vi "Logging Message Loop.vi"(8 "error in (no error)":errorcluster, 10 "Data Queue":T1, 11 "Message Queues":T2) -> (0 "error out":errorcluster)   [LabVIEW 2015, in "Logging.lvlib"]
doc: "The message loop subVI to handle messages pertaining to logging data."
uses:
  Logging.lvlib
  Support VIs/Message Queue/All Message Queues.ctl
  Support VIs/Message Queue/Message Cluster.ctl
  controls/Data queue.ctl
  Acquisition/Generic data packet.ctl
  My Graphs/Gps Map Graph coordinates.ctl
  Logging Configuration.ctl
  Logging State.ctl
  Support VIs/Message Queue/Enqueue Message (Single).vi
  <vilib>/Utility/error.llb/Error Cluster From Error Code.vi
  <vilib>/ErrorRing/Error Ring.xnode
  Support VIs/Message Queue/Message Queue.lvlib
  Acquisition/Acquisition.lvlib
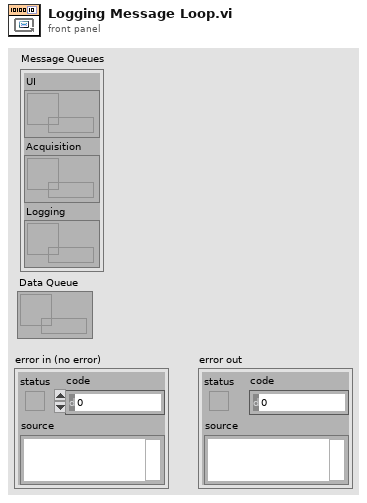
[diagram p1: front panel]
types:
  T1 = typedef "Data queue.ctl" = refnum<queue>
  T2 = typedef "Message Queue.lvlib/All Message Queues.ctl" = cluster{"UI":refnum<queue>, "Acquisition":refnum<queue>, "Logging":refnum<queue>}
  T3 = typedef "Logging.lvlib/Logging Configuration.ctl" = cluster{"Log File Base Path":path, "TDMS File Reference":refnum<k34>, "Data format":enum16{"IDRA data", "XAM data"}}
  T4 = cluster{"log_number":i32, "log_timestamp":string}
  T5 = typedef "Logging.lvlib/Logging State.ctl" = enum16{"Idle", "Logging"}
  T6 = enum16{"open", "open or create", "create or replace", "create", "open (read-only)"}
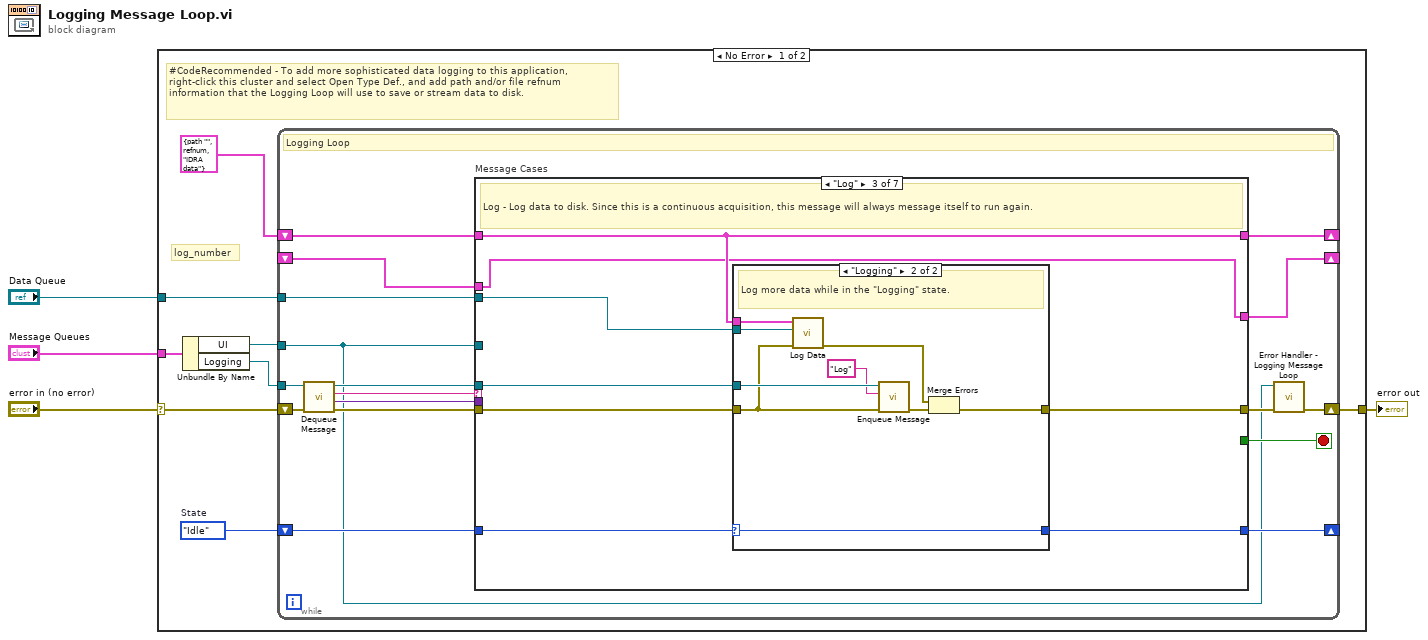
[diagram p0: block diagram]
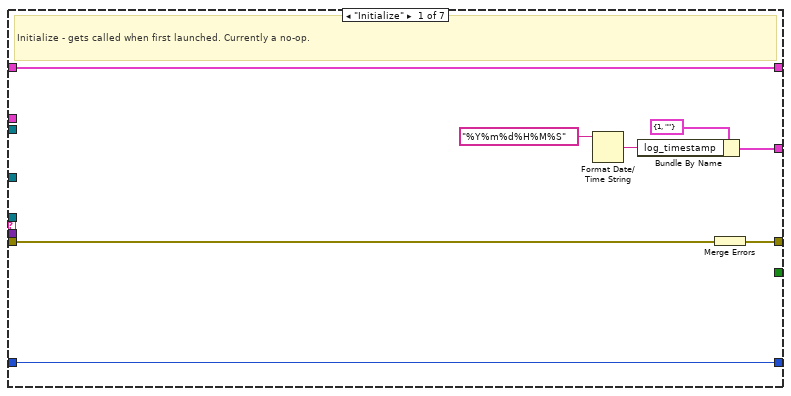
[diagram p2: hidden frame]
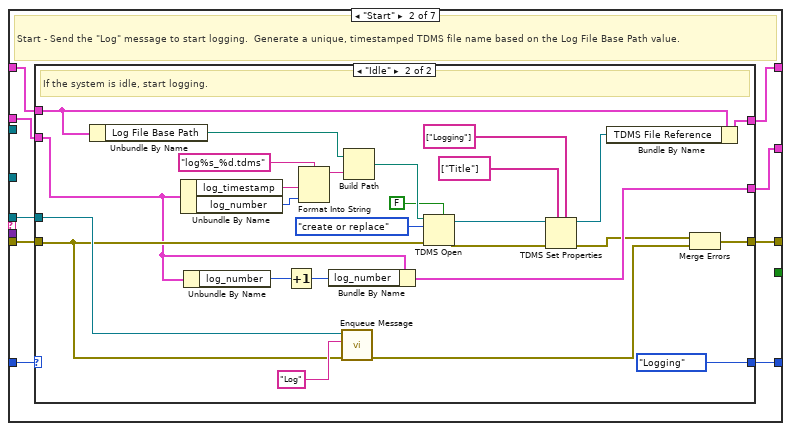
[diagram p3: hidden frame]
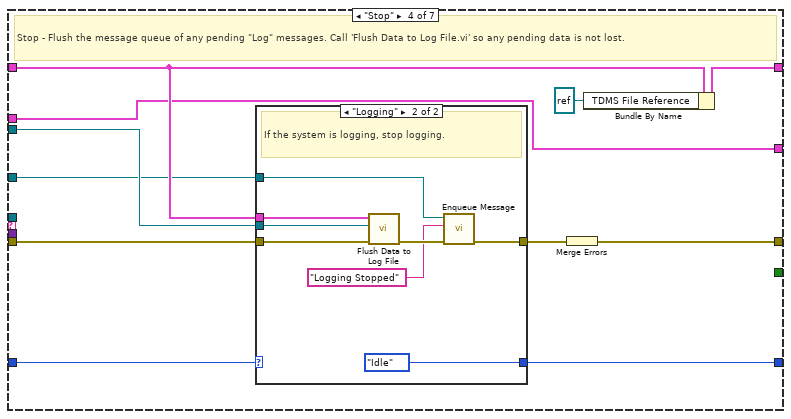
[diagram p6: hidden frame]
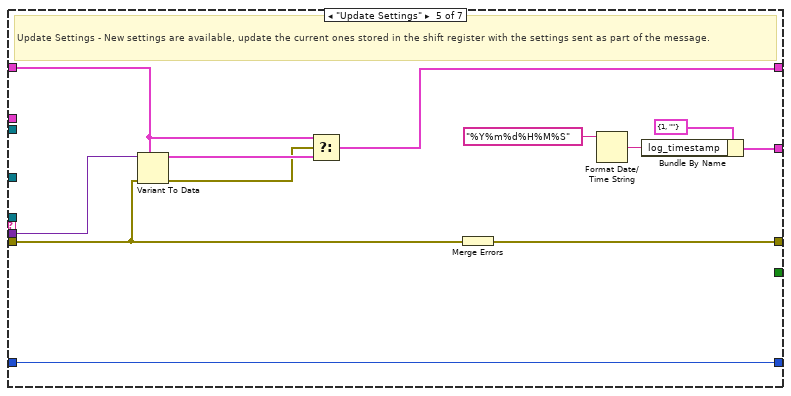
[diagram p8: hidden frame]
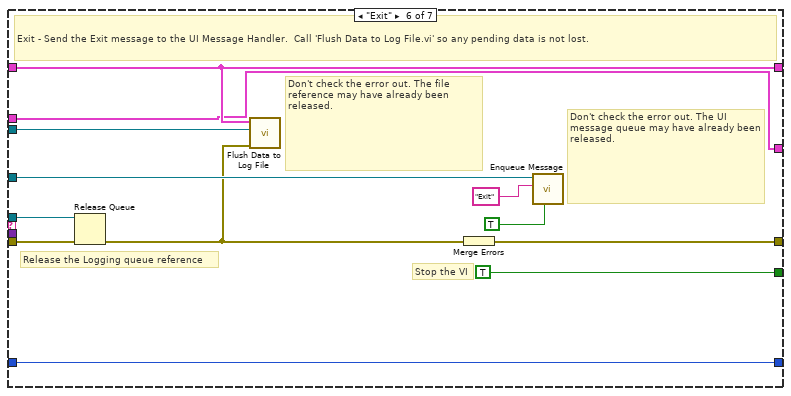
[diagram p9: hidden frame]
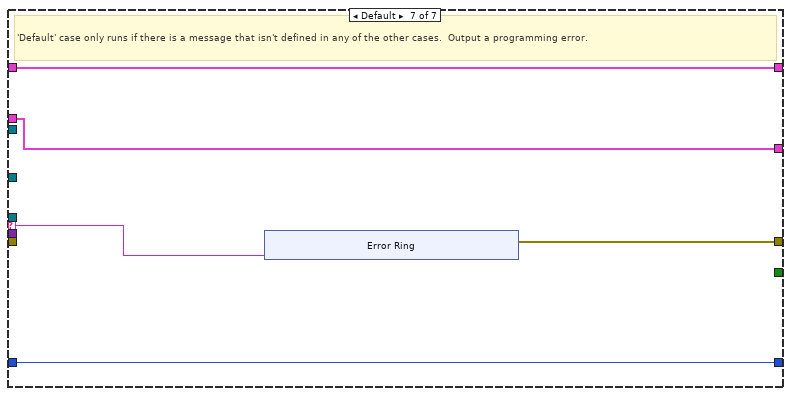
[diagram p10: hidden frame]
diagram:
  n1 = case shown="No Error" "error in (no error)" {
    selector: "error in (no error)" -> [w8 w153]
    tunnel: "Message Queues" -> [w12 _]
    tunnel: [w10 w153] -> w3
    tunnel: "Data Queue" -> [w7 _]
    frame No Error {
      w5 = Logging_State."Idle"  # State
      # "log_number"
      # "#CodeRecommended - To add more sophisticated data logging to this application, right-click this cluster and select Open Type Def., and add path and/or file refnum information that the Logging Loop will use to save or stream data to disk."
      n2 = Unbundle By Name(w12) -> ("UI"=w6:refnum<queue>, "Logging"=w11:refnum<queue>)
      n3 = while {
        tunnel: w11 -> [w21]
        shift-right: [w28] -> _
        shift-left: T3 {"Log File Base Path"=path "", "TDMS File Reference"=refnum, "Data format"=enum."IDRA data"} ("Logging Configuration") -> [w29]
        shift-right: [w17] -> w10
        shift-left: w8 -> [w26]
        tunnel: w6 -> [w15]
        tunnel: w7 -> [w20]
        shift-right: [w18] -> _
        shift-left: w5 -> [w19]
        shift-right: [w14] -> _
        shift-left: _ -> [w13]
        stop <- w27 stop-if-true
        # "Logging Loop"
        n4 = call "Dequeue Message.vi"("error in (no error)"=w26, "Message Queue"=w21) -> ("error out"=w25:errorcluster, "Message Data"=w23:variant, "Message"=w24:string, "dup Message Queue"=w22:refnum<queue>)  [unwired: 6 in]
        n5 = case "Message Cases" shown="\"Log\"" w24 {
          selector: w24 -> [_ _ _ _ _ _ w142]
          tunnel: w22 -> [_ w45 w83 _ _ w134 _]
          tunnel: w25 -> [w35 w44 w81 w100 w122 w137 _]
          tunnel: [w37 w46 w84 w106 w128 w139 w143] -> w16
          tunnel: w29 -> [w36 w43 w80 w101 w126 w132 w145]
          tunnel: [w36 w42 w80 w104 w123 w132 w145] -> w28
          tunnel: [_ _ _ _ _ TRUE _] -> w27
          tunnel: w23 -> [_ _ _ _ w127 _ _]
          tunnel: w15 -> [_ _ _ w97 _ w138 _]
          tunnel: w20 -> [_ _ w82 w102 _ w131 _]
          tunnel: w19 -> [w34 w41 w79 w99 w121 w130 w144]
          tunnel: [w34 w40 w78 w98 w121 w130 w144] -> w18
          tunnel: [w30 w38 w77 w96 w119 w129 w141] -> w14
          tunnel: w13 -> [_ w39 w77 w96 _ w129 w141]
          frame "Initialize" {
            # "Initialize - gets called when first launched. Currently a no-op."
            n6 = Format Date/Time String(time format string (%c)="%Y%m%d%H%M%S") -> (date/time string=w31:string)  [unwired: 2 in]
            n7 = Bundle By Name(cluster=T4 {"log_number"=1, "log_timestamp"=""}, "log_timestamp"=w31) -> (w30:T4)
            n8 = Merge Errors(w35) -> (w37:errorcluster)
          }
          frame "Start" {
            # "Start - Send the \"Log\" message to start logging.  Generate a unique, timestamped TDMS file name based on the Log File Base Path value."
            n9 = case shown="\"Idle\"" w41 {
              selector: w41 -> [w49 _]
              tunnel: [w48 w67] -> w46
              tunnel: w45 -> [_ w68]
              tunnel: w44 -> [w48 w66]
              tunnel: w43 -> [w50 w69]
              tunnel: [w50 w71] -> w42
              tunnel: [w49 Logging_State."Logging" ("State")] -> w40
              tunnel: w39 -> [w47 w61]
              tunnel: [w47 w58] -> w38
              frame "Logging" {
                # "The system is already logging. Ignore the \"Start\" message."
              }
              frame "Idle" {
                # "If the system is idle, start logging."
                n10 = Unbundle By Name(w69) -> ("Log File Base Path"=w65:path)
                n11 = Unbundle By Name(w61) -> ("log_timestamp"=w63:string, "log_number"=w62:i32)
                n12 = Unbundle By Name(w61) -> ("log_number"=w60:i32)
                n13 = Increment(x=w60) -> (x+1=w59:i32)
                n14 = Format Into String(format string="log%s_%d.tdms", w63, w62) -> (resulting string=w74:string)  [unwired: 2 in, 1 out]
                n15 = Bundle By Name(cluster=w61, "log_number"=w59) -> (w58:T4)
                n16 = call-poly "Enqueue Message.vi"("error in (no error)"=w66, "Message"="Log", "Message Queue"=w68) -> ("error out"=w64:errorcluster)  [unwired: 7 in, 1 out]
                n17 = Build Path(base path=w65, name or relative path=w74) -> (appended path=w73:path)
                n18 = TDMS Open(5:FALSE ("create index file? (T)"), 8:w66, 10:T6."create or replace" ("operation (0:open)"), 11:w73) -> (0:w56:errorcluster, 3:w53:refnum<k34>)  [unwired: 3 in]
                n19 = TDMS Set Properties(5:string[] ["Logging"] ("property values"), 7:string[] ["Title"] ("property names"), 8:w56, 11:w53) -> (0:w55:errorcluster, 3:w54:refnum<k34>)  [unwired: 2 in, 2 out]
                n20 = Bundle By Name(cluster=w69, "TDMS File Reference"=w54) -> (w71:T3)
                n21 = Merge Errors(w55, w64) -> (w67:errorcluster)
              }
            }
          }
          frame "Log" {
            # "Log - Log data to disk. Since this is a continuous acquisition, this message will always message itself to run again."
            n22 = case shown="\"Logging\"" w79 {
              selector: w79 -> [w86 w88]
              tunnel: [w85 w95] -> w84
              tunnel: w83 -> [_ w93]
              tunnel: w82 -> [_ w92]
              tunnel: w81 -> [w85 w87]
              tunnel: w80 -> [_ w89]
              tunnel: [w86 w88] -> w78
              frame "Idle" {
                # "Ignore \"Log\" messages when the logging is idle."
              }
              frame "Logging" {
                # "Log more data while in the \"Logging\" state."
                n23 = call "Log Data.vi"("error in (no error)"=w87, "Data Queue"=w92, "Logging Configuration"=w89) -> ("error out"=w91:errorcluster)  [unwired: 8 in]
                n24 = call-poly "Enqueue Message.vi"("error in (no error)"=w87, "Message"="Log", "Message Queue"=w93) -> ("error out"=w94:errorcluster)  [unwired: 7 in, 1 out]
                n25 = Merge Errors(w91, w94) -> (w95:errorcluster)
              }
            }
          }
          frame "Stop" {
            # "Stop - Flush the message queue of any pending \"Log\" messages. Call 'Flush Data to Log File.vi' so any pending data is not lost."
            n26 = case shown="\"Logging\"" w99 {
              selector: w99 -> [w107 _]
              tunnel: [w108 w111] -> w105
              tunnel: w102 -> [_ w115]
              tunnel: w101 -> [_ w114]
              tunnel: w100 -> [w108 w113]
              tunnel: [w107 Logging_State."Idle" ("State")] -> w98
              tunnel: w97 -> [_ w110]
              frame "Idle" {
                # "The system is already idle. Ignore the \"Stop\" message."
              }
              frame "Logging" {
                # "If the system is logging, stop logging."
                n27 = call "Flush Data to Log File.vi"("error in (no error)"=w113, "Data Queue"=w115, "Logging Configuration"=w114) -> ("error out"=w116:errorcluster)  [unwired: 8 in]
                n28 = call-poly "Enqueue Message.vi"("error in (no error)"=w116, "Message"="Logging Stopped", "Message Queue"=w110) -> ("error out"=w111:errorcluster)  [unwired: 7 in, 1 out]
              }
            }
            n29 = Merge Errors(w105) -> (w106:errorcluster)
            n30 = Bundle By Name(cluster=w101, "TDMS File Reference"=refnum<k34> refnum) -> (w104:T3)
          }
          frame "Update Settings" {
            # "Update Settings - New settings are available, update the current ones stored in the shift register with the settings sent as part of the message."
            n31 = Variant To Data(error in=w122, type=w126, Variant=w127) -> (data=w125:T3, error out=w124:errorcluster)
            n32 = Select(t=w126, s=w124, f=w125) -> (s? t:f=w123:T3)
            n33 = Merge Errors(w122) -> (w128:errorcluster)
            n34 = Format Date/Time String(time format string (%c)="%Y%m%d%H%M%S") -> (date/time string=w117:string)  [unwired: 2 in]
            n35 = Bundle By Name(cluster=T4 {"log_number"=1, "log_timestamp"=""}, "log_timestamp"=w117) -> (w119:T4)
          }
          frame "Exit" {
            # "Don't check the error out. The file reference may have already been released."
            # "Release the Logging queue reference"
            # "Don't check the error out. The UI message queue may have already been released."
            # "Stop the VI"
            # "Exit - Send the Exit message to the UI Message Handler.  Call 'Flush Data to Log File.vi' so any pending data is not lost."
            n36 = Release Queue(queue=w134, error in (no error)=w137) -> (error out=w133:errorcluster)  [unwired: 1 in, 2 out]
            n37 = call "Flush Data to Log File.vi"("error in (no error)"=w133, "Data Queue"=w131, "Logging Configuration"=w132) -> ()  [unwired: 8 in, 1 out]
            n38 = Merge Errors(w133) -> (w139:errorcluster)
            n39 = call-poly "Enqueue Message.vi"("Priority Message? (F)"=TRUE, "Message"="Exit", "Message Queue"=w138) -> ()  [unwired: 7 in, 2 out]
          }
          frame Default {
            # "'Default' case only runs if there is a message that isn't defined in any of the other cases.  Output a programming error."
            n40 = xnode "Error Ring"("parameter 0"=w142) -> ("error out"=w143:errorcluster)
          }
        }
        n41 = call "Error Handler - Logging Message Loop.vi"("error in (no error)"=w16, "Message Queue"=w15) -> ("dup error in"=w17:errorcluster)  [unwired: 8 in, 1 out]
      }
    }
    frame Error {
    }
  }
  "error out" <- w3
